vi "start_delay_autocorrect_rrMD.vi"   [LabVIEW 2012]
doc: "SciScan 1.2 160622"
uses:
  GFG/GFGbooleanGet.vi
  GFG/GFGnumericGet.vi
  GFG/GFGImageRefsGet.vi
  GFG/GFGfpRefGet.vi
  GFG/GFG library.lvlib
  <vilib>/vision/NI_Vision_Development_Module.lvlib
types:
  T1 = enum32{"Channel 1", "Channel 2", "Channel 3", "Channel 4", "Channel 5", "all channels", "RGB overlay", "ROI", "arbitrary line scan"}
  T2 = typedef "IMAQ Image.ctl" = refnum<image>
  T3 = cluster{"Channel 1 small":T2, "Channel 2 small":T2, "Channel 3 small":T2, "Channel 4 small":T2, "Channel 1 large":T2, "Channel 2 large":T2, "Channel 3 large":T2, "Channel 4 large":T2, "RGB overlay":T2, "ROI Image display":T2, "arb line scan display":T2, "Channel 5 large":T2}
  T4 = typedef "Image Type" = u32
  T5 = cluster{"WaveformChartRef":refnum<vi>, "DigitalRef":refnum<vi>, "ArrayRef":refnum<vi>, "TabControlRef":refnum<vi>, "EnumRef":refnum<vi>, "RingRef":refnum<vi>, "BooleanRef":refnum<vi>, "KnobRef":refnum<vi>, "SlideRef":refnum<vi>, "PathRef":refnum<vi>, "StringRef":refnum<vi>, "ComboBox":refnum<vi>, "WaveformGraphRef":refnum<vi>}
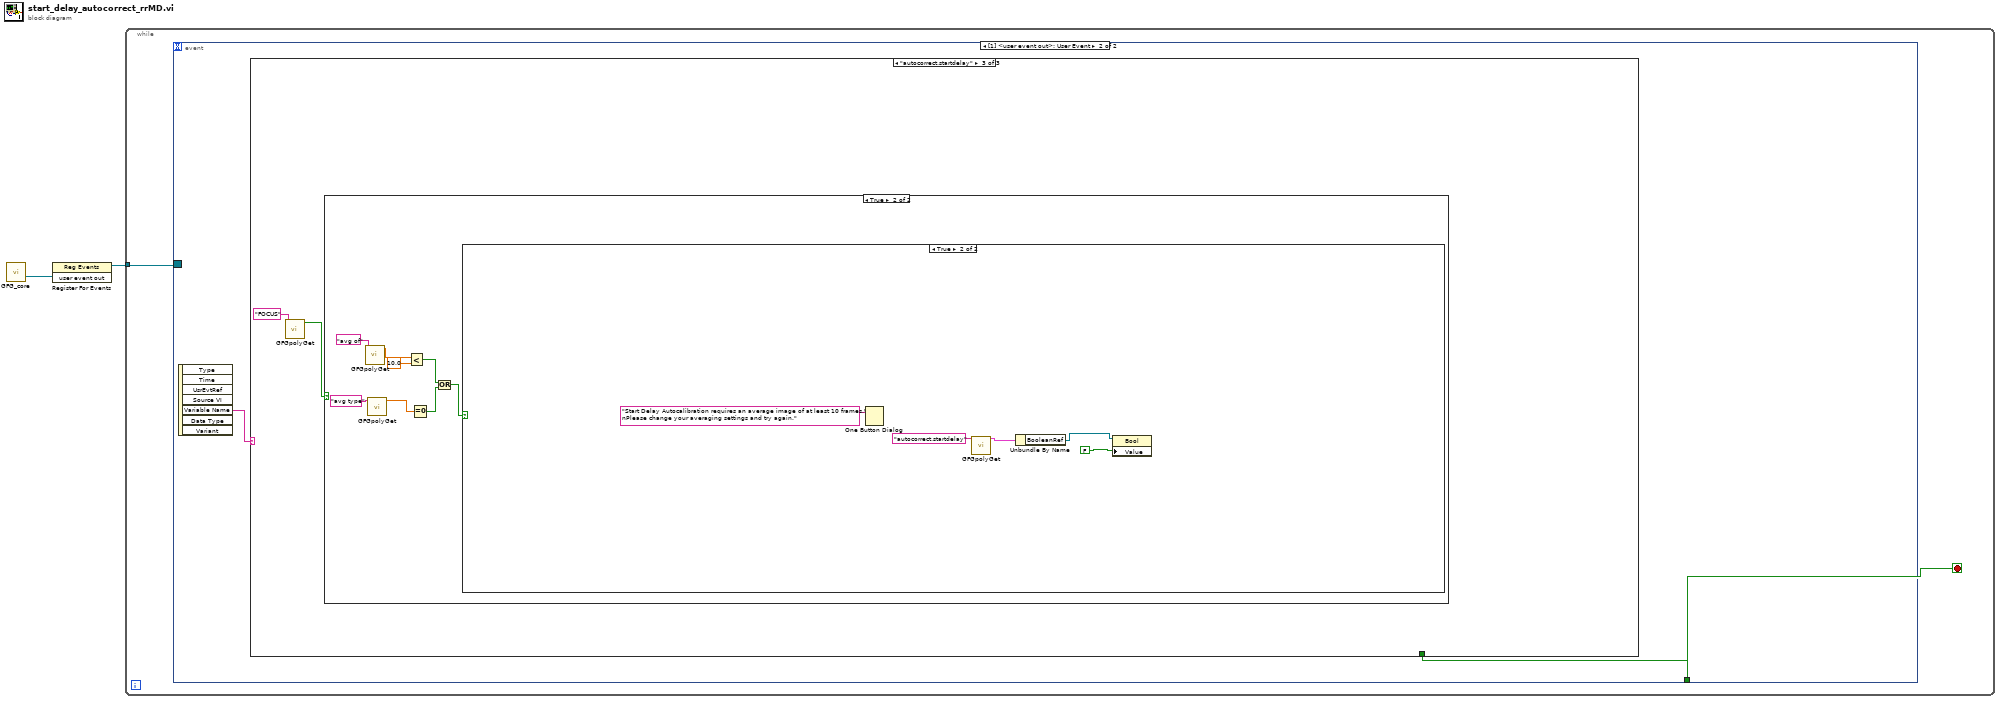
[diagram p0: block diagram]
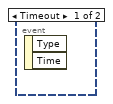
[diagram p2: hidden frame]
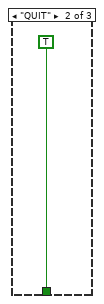
[diagram p4: hidden frame]
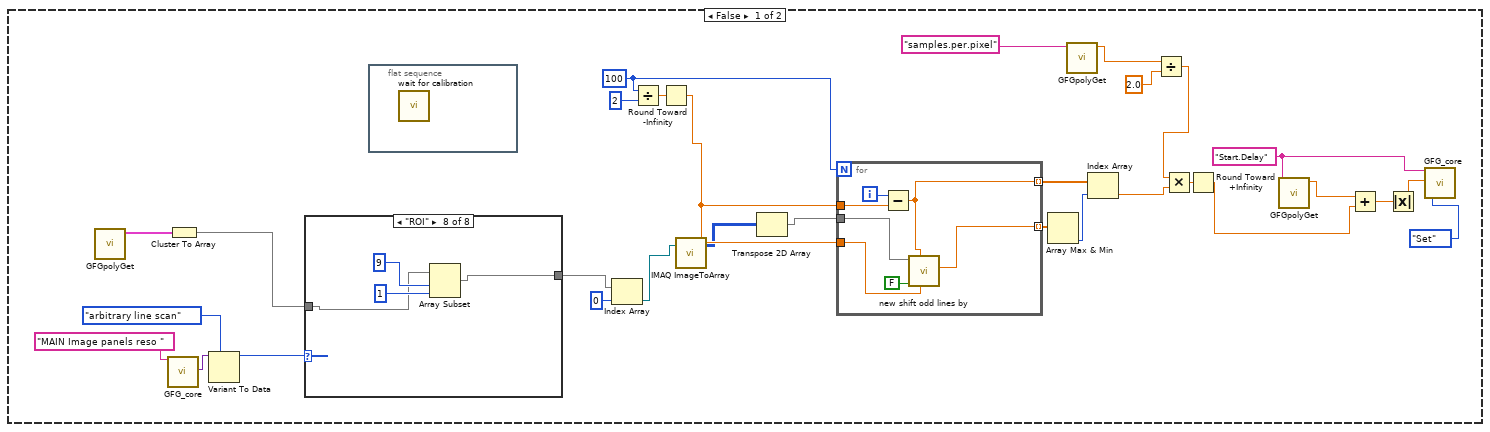
[diagram p6: hidden frame]
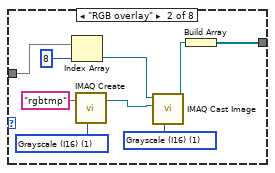
[diagram p8: hidden frame]
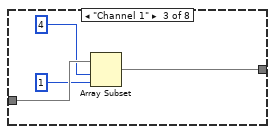
[diagram p9: hidden frame]
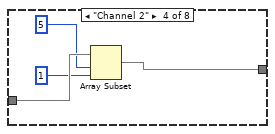
[diagram p10: hidden frame]
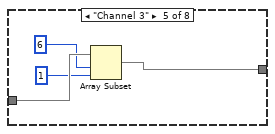
[diagram p11: hidden frame]
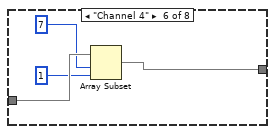
[diagram p12: hidden frame]
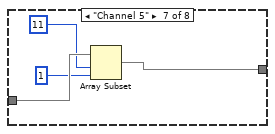
[diagram p13: hidden frame]
diagram:
  n1 = call "GFG_core.vi"() -> ("user event out"=w2:refnum<user-event>)  [unwired: 13 in, 6 out]
  n2 = register-events(w2) -> (reference out=w1:refnum<event-registration>)  [unwired: 2 in, 1 out]
  n3 = while {
    tunnel: w1 -> [w4]
    stop <- w3 stop-if-true
    n4 = event shown="[1] <user event out>: User Event" {
      selector: w4 -> [_ _]
      dyn-events: _ -> [_ _]
      timeout: _ -> [_ _]
      tunnel: [_ w5] -> w3
      event Timeout {
        n5 = event-data() -> ()  [unwired: 1 in, 2 out]
      }
      event User Event {
        n6 = event-data() -> ("Variable Name"=w6:string)  [unwired: 1 in, 6 out]
        n7 = case shown="\"autocorrect.startdelay\"" w6 {
          tunnel: [_ TRUE _] -> w5
          frame "False", Default {
          }
          frame "QUIT" {
          }
          frame "autocorrect.startdelay" {
            n8 = call-poly "GFGpolyGet.vi"("Variable Name in"="FOCUS") -> ("Boolean Value OUT"=w8:bool)  [unwired: 9 in, 1 out]
            n9 = case shown="True" w8 {
              frame False {
              }
              frame True {
                n10 = call-poly "GFGpolyGet.vi"("Variable Name in"="avg of") -> ("Numeric"=w14:dbl)  [unwired: 8 in, 2 out]
                n11 = call-poly "GFGpolyGet.vi"("Variable Name in"="avg type") -> ("Numeric"=w15:dbl)  [unwired: 8 in, 2 out]
                n12 = Less?(x=w14, y=10.0) -> (x < y?=w12:bool)
                n13 = Equal To 0?(x=w15) -> (x = 0?=w11:bool)
                n14 = Or(x=w12, y=w11) -> (x .or. y?=w10:bool)
                n15 = case shown="True" w10 {
                  frame False {
                    w29 = "Start.Delay" ("Variable Name in")
                    w22 = 100 ("Numeric")
                    n16 = call-poly "GFGpolyGet.vi"() -> ("Image Refs Out"=w34:T3)  [unwired: 10 in, 1 out]
                    n17 = call "GFG_core.vi"("Variable Name in"="MAIN Image panels reso ") -> ("Variant Out"=w37:variant)  [unwired: 12 in, 6 out]
                    n18 = Cluster To Array(cluster=w34) -> (array=w33:T2[])
                    n19 = Variant To Data(type=T1."arbitrary line scan" ("MAIN Image panels"), Variant=w37) -> (data=w35:T1)  [unwired: 1 in, 1 out]
                    n20 = case shown="\"ROI\"" w35 {
                      tunnel: w33 -> [_ w56 w60 w64 w68 w72 w76 w78]
                      tunnel: [_ w48 w57 w61 w65 w69 w73 w77] -> w32
                      frame Default {
                      }
                      frame "RGB overlay" {
                        w50 = T4 1 items=["Grayscale (U8)", "Grayscale (I16)", "Grayscale (SGL)", "Complex (CSG)", "RGB (U32)", "HSL (U32)", "RGB (U64)", "Grayscale (U16)"] ("Image Type")
                        w53 = T4 1 items=["Grayscale (U8)", "Grayscale (I16)", "Grayscale (SGL)", "Complex (CSG)", "RGB (U32)", "HSL (U32)", "RGB (U64)", "Grayscale (U16)"] ("Image Type")
                        n21 = Index Array(array=w56, index=8) -> (element=w51:T2)
                        n22 = call "IMAQ Create"("Image Name"="rgbtmp", "Image Type"=w53) -> ("New Image"=w52:T2)  [unwired: 3 in, 1 out]
                        n23 = call "IMAQ Cast Image"("Image Type"=w50, "Image Dst"=w52, "Image Src"=w51) -> ("Image Dst Out"=w49:T2)  [unwired: 7 in, 1 out]
                        n24 = Build Array(w49) -> (w48:T2[])
                      }
                      frame "Channel 1" {
                        n25 = Array Subset(array=w60, index=4, length=1) -> (w57:T2[])
                      }
                      frame "Channel 2" {
                        n26 = Array Subset(array=w64, index=5, length=1) -> (w61:T2[])
                      }
                      frame "Channel 3" {
                        n27 = Array Subset(array=w68, index=6, length=1 ("index")) -> (w65:T2[])
                      }
                      frame "Channel 4" {
                        n28 = Array Subset(array=w72, index=7, length=1 ("index")) -> (w69:T2[])
                      }
                      frame "Channel 5" {
                        n29 = Array Subset(array=w76, index=11, length=1 ("index")) -> (w73:T2[])
                      }
                      frame "ROI" {
                        n30 = Array Subset(array=w78, index=9, length=1 ("index")) -> (w77:T2[])
                      }
                    }
                    n31 = flat-sequence {
                      frame #0 {
                        n32 = call "wait for calibration.vi"() -> ()  [unwired: 12 in]
                      }
                    }
                    n33 = Index Array(array=w32, index=0) -> (element=w20:T2)
                    n34 = Divide(x=w22, y=2) -> (x/y=w46:dbl)
                    n35 = Round Toward -Infinity(1:w46) -> (0:w21:dbl)
                    n36 = call "IMAQ ImageToArray"("Image"=w20) -> ("Image Pixels (I16)"=w19:i16[][])  [unwired: 3 in, 4 out]
                    n37 = Transpose 2D Array(2D array=w19) -> (transposed array=w18:i16[][])
                    n38 = for {
                      N: w22 -> [_]
                      tunnel: w18 -> [w84]
                      tunnel: w21 -> [w87]
                      tunnel: [w82] -> w45 mode=indexing
                      tunnel: [w83] -> w43 mode=indexing
                      tunnel: w21 -> [w85]
                      i -> [w86]
                      n39 = Subtract(x=w86, y=w87) -> (x-y=w83:dbl)
                      n40 = call "new shift odd lines by.vi"("max pix shift"=w85, "shift odd lines by"=w83, "calculate shited frame"=FALSE, "pixel array in (x is first dimension)"=w84) -> ("squared difference"=w82:dbl)  [unwired: 6 in, 1 out]
                    }
                    n41 = Array Max & Min(array=w45) -> (min index (indices)=w44:i32)  [unwired: 3 out]
                    n42 = call-poly "GFGpolyGet.vi"("Variable Name in"="samples.per.pixel") -> ("Numeric"=w25:dbl)  [unwired: 8 in, 2 out]
                    n43 = Index Array(array=w43, index=w44) -> (element=w42:dbl)
                    n44 = Divide(x=w25, y=2.0) -> (x/y=w24:dbl)
                    n45 = Multiply(x=w24, y=w42) -> (x*y=w41:dbl)
                    n46 = Round Toward +Infinity(x=w41) -> (ceil(x): smallest int >= x=w39:dbl)
                    n47 = call-poly "GFGpolyGet.vi"("Variable Name in"=w29) -> ("Numeric"=w40:dbl)  [unwired: 8 in, 2 out]
                    n48 = Add(x=w40, y=w39) -> (x+y=w28:dbl)
                    n49 = Absolute Value(x=w28) -> (abs(x)=w27:dbl)
                    n50 = call "GFG_core.vi"("Variable Name in"=w29, "Variant in"=w27, "Action"=enum16{"Init", "Set", "Get"}."Set") -> ()  [unwired: 10 in, 7 out]
                  }
                  frame True {
                    n51 = One Button Dialog(message="Start Delay Autocalibration requires an average image of at least 10 frames.\nPlease change your averaging settings and try again.") -> ()  [unwired: 1 in, 1 out]
                    n52 = call-poly "GFGpolyGet.vi"("Variable Name in"="autocorrect.startdelay") -> ("output cluster"=w91:T5)  [unwired: 9 in, 1 out]
                    n53 = Unbundle By Name(w91) -> ("BooleanRef"=w89:refnum<vi>)
                    n54 = property class="Bool"(reference=w89, "Value"=FALSE ("x .or. y?")) -> ()  [unwired: 1 in, 2 out]
                  }
                }
              }
            }
          }
        }
      }
    }
  }
